vi "LDA_global.vi"() -> ()   [LabVIEW 2022 SP3]
uses:
  LDA/BSA_With_IP/LDA_Channel.ctl
  Controls/Correlation_cluster1.ctl
panel:
  out "Connected Laser Dx number":i64[](array[numeric])
  out "Laser Connect error out":errorcluster
  out "Connected Laser Dx Refs":refnum<k7>[](array[refnum])
  in  "Laser IP Number":string="10.10.100.130"
  in  "Connected Laser Dx IPs":string[](array[string])
  in  "Available Laser Dx IP Numbers":string[](array[string])
  in  "Connect Laser Dx":refnum<k4>
  in  "Available Laser Dx names":string[](array[string])
  out "3DLDA Correlations":T1[](array[typedef]) {"Time Window (ms)" format="%.2f"; "w^2 Paired" format="%.2f"; "u^2 Paired" format="%.2f"; "u^2w^2" format="%.2f"; "u^3w" format="%.2f"; "uw^3" format="%.2f"; "uw/u'w'" format="%.2f"; "uw^2" format="%.2f"; "u^2w" format="%.2f"; "uw" format="%.2f"}
  out "Connect error out":errorcluster
  out "Connected BSA References":refnum<k7>[](array[refnum])
  in  "Connected BSA IPs":string[](array[string])
  in  "BSA IP Number":string="10.10.100.130"
  in  "Connect BSA":refnum<k4>
  in  "Non-coincident":bool
  in  "Older LDA Data":dbl[][](array[numeric])
  out "LDA Raw Data":cluster{dbl[][]}[](array[cluster])
  in  "Number of LDA Chs":i32 min=0 max=20
  in  "LDA Channels":T2[](array[typedef]) {"Sync Delay (s)" format="%.2g"; "Req Sampling Rate Hz" min=1.0; "Shifted mW" format="%.1g"; "Unshifted mW" format="%.1g"; "Centre Velocity (m/s)" format="%.2g"; "Velocity Range (m/s)" format="%.2g"; "Focal Length (mm)" format="%.1f"; "Beam Separation (mm)" format="%.1f"; "Optics Conversion Factor" format="%.3g"; "High voltage" min=0 max=2040 step=8; "Signal gain (dB)" min=0 max=30 step=1; "Min Velocity" format="%.2g"; "Max Velocity" format="%.2g"; "Wavelength (nm)" format="%.1f"}
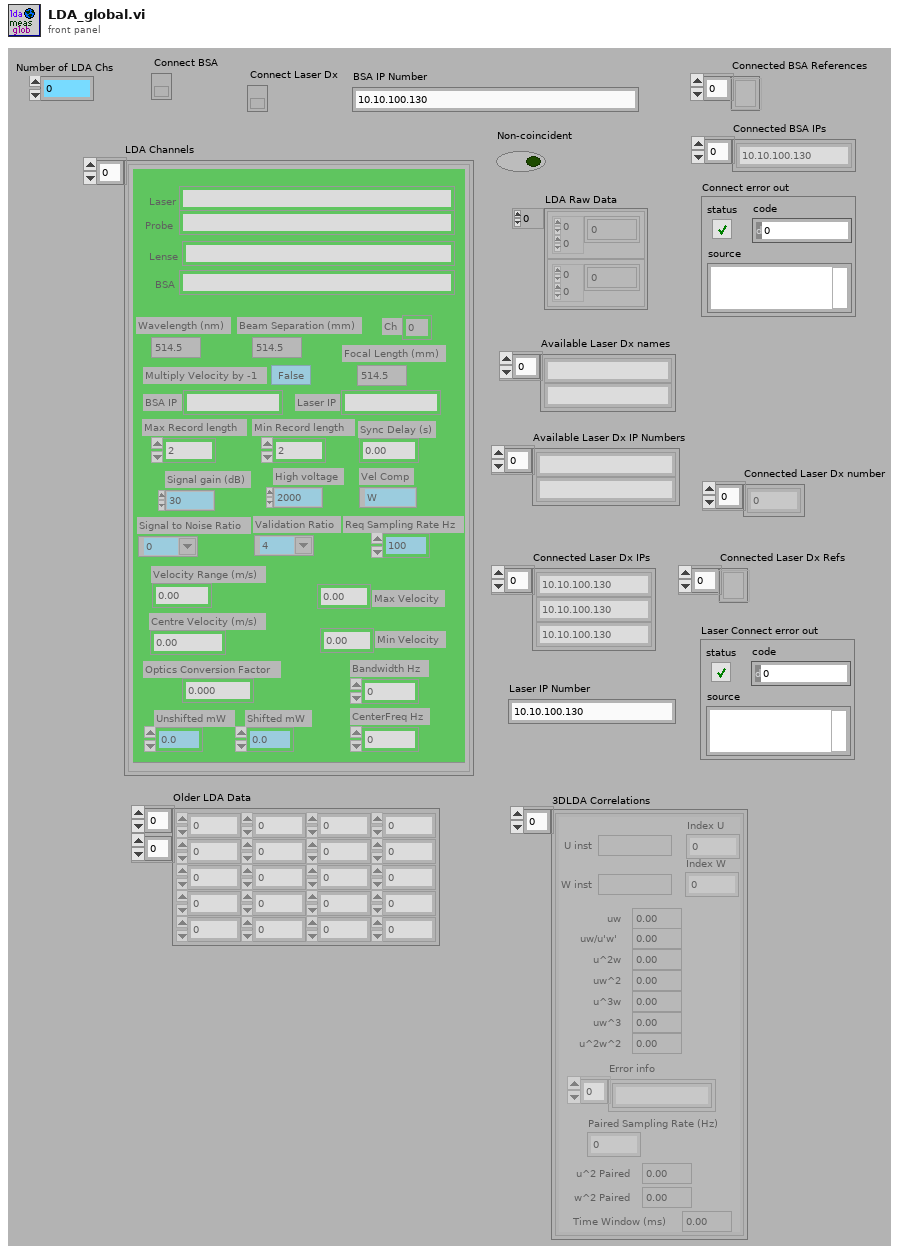
[diagram p1: front panel]
types:
  T1 = typedef "Correlation_cluster1.ctl" = cluster{"U inst":string, "uw":dbl, "u^2w":dbl, "uw^2":dbl, "uw/u'w'":dbl, "W inst":string, "uw^3":dbl, "u^3w":dbl, "u^2w^2":dbl, "Index U":i32, "Index W":i32, "Error info":string[], "Paired Sampling Rate (Hz)":dbl, "u^2 Paired":dbl, "w^2 Paired":dbl, "Time Window (ms)":dbl}
  T2 = typedef "LDA_Channel.ctl" = cluster{"Wavelength (nm)":dbl, "Vel Comp":string, "Max Velocity":dbl, "Min Velocity":dbl, "Max Record length":u16, "Signal gain (dB)":i16, "High voltage":i16, "Optics Conversion Factor":dbl, "Min Record length":u16, "Multiply Velocity by -1":bool, "Signal to Noise Ratio":string, "Validation Ratio":string, "Probe":string, "Laser":string, "BSA":string, "Lense":string, "Beam Separation (mm)":dbl, "Focal Length (mm)":dbl, "COLOUR":u32, "BSA IP":string, "Velocity Range (m/s)":dbl, "Centre Velocity (m/s)":dbl, "Unshifted mW":dbl, "Shifted mW":dbl, "Bandwidth Hz":dbl, "Req Sampling Rate Hz":dbl, "Ch":i32, "CenterFreq Hz":dbl, "Laser IP":string, "Sync Delay (s)":dbl}
diagram:
